vi "Send Configure Stop Trigger [SPT].vi"(6 "Trigger Slope (Positive)":i32(ring) caption="trigger slope (Positive)" items=["Positive", "Negative", "Either"], 7 "Message Priority (Normal)":T1=enum."Normal", 8 "error in (no error)":errorcluster, 9 "Trigger Source (None)":string(combo) caption="trigger source (None)", 10 "Channel Name (\"\")":string="CHANNEL1" caption="channel name (\"CHANNEL1\")", 11 "Message Enqueuer":refnum<class "Message Enqueuer.lvclass">) -> (0 "error out":errorcluster, 3 "Message Enqueuer out":refnum<class "Message Enqueuer.lvclass">)   [LabVIEW 2015, in "CS++Fgen.lvlib" / "Configure Stop Trigger [SPT] Msg.lvclass"]
doc: "Sends the <B>CS++Fgen.lvlib:Configure Stop Trigger [SPT] Msg.lvclass</B> message.\n\n<B>CS++Fgen.lvlib:CS++Fgen.lvclass:Configure Stop Trigger [SPT].vi</B> Description:\n\nThis VI configures the properties that control the function generator's stop trigger. These properties are the stop trigger source and slope.\n\nA stop trigger terminates any generation and has the same effect as calling the IviFgen Abort Generation VI.\n\nNote:\n\n(1) This VI is part of the IviFgenStopTrigger [SPT] extension group."
uses:
  Configure Stop Trigger [SPT] Msg.lvclass
  <vilib>/ActorFramework/Message Enqueuer/Message Enqueuer.lvclass
  <vilib>/ActorFramework/Message Enqueuer/Message Priority.ctl
  Configure Stop Trigger [SPT] Msg.lvclass/Configure Stop Trigger [SPT] Msg.ctl
  <vilib>/ActorFramework/Message Enqueuer/Message Enqueuer.lvclass/Message Enqueuer.ctl
  <vilib>/ActorFramework/Message Priority Queue/Priority Enqueue.vi
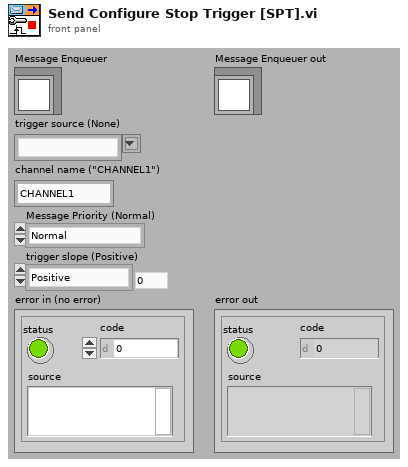
[diagram p1: front panel]
types:
  T1 = typedef "Actor Framework.lvlib/Message Enqueuer.lvclass/Message Priority.ctl" = enum16{"Low", "Normal", "High"}
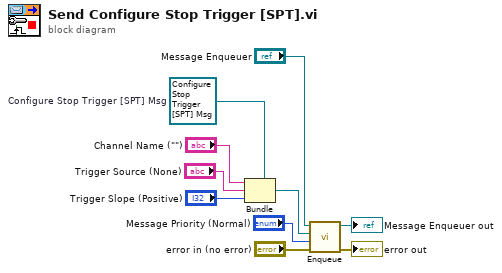
[diagram p0: block diagram]
diagram:
  w4 = refnum<class "Configure Stop Trigger [SPT] Msg.lvclass"> refnum  # Configure Stop Trigger [SPT] Msg
  n1 = Bundle(cluster=w4, "Channel Name (\"\")", "Trigger Source (None)", "Trigger Slope (Positive)") -> (w7:refnum<class "Configure Stop Trigger [SPT] Msg.lvclass">)
  n2 = call <vilib>:"Enqueue.vi"("error in (no error)"="error in (no error)", "Message Priority (Normal)"="Message Priority (Normal)", "Message"=w7, "Message Enqueuer in"="Message Enqueuer") -> ("error out"=→"error out":errorcluster, "Message Enqueuer out"=→"Message Enqueuer out":refnum<class "Message Enqueuer.lvclass">)  [unwired: 6 in]
